vi "Upload_Balance Data_to_Server.vi"() -> ()   [LabVIEW 2015]
uses:
  Controls/Post_Process.ctl
  Globals/Meas_global.vi
panel:
  in  "millisecond multiple":dbl=100.0
  out "roll":dbl(graph)
  out "yaw":dbl(graph)
  out "side":dbl(graph)
  out "drag":dbl(graph)
  out "pitch":dbl(graph)
  out "lift":dbl(graph)
  out "appended array":dbl[](array[numeric])
  out "Monitor Speed (Hz)":dbl
  in  "stop":bool
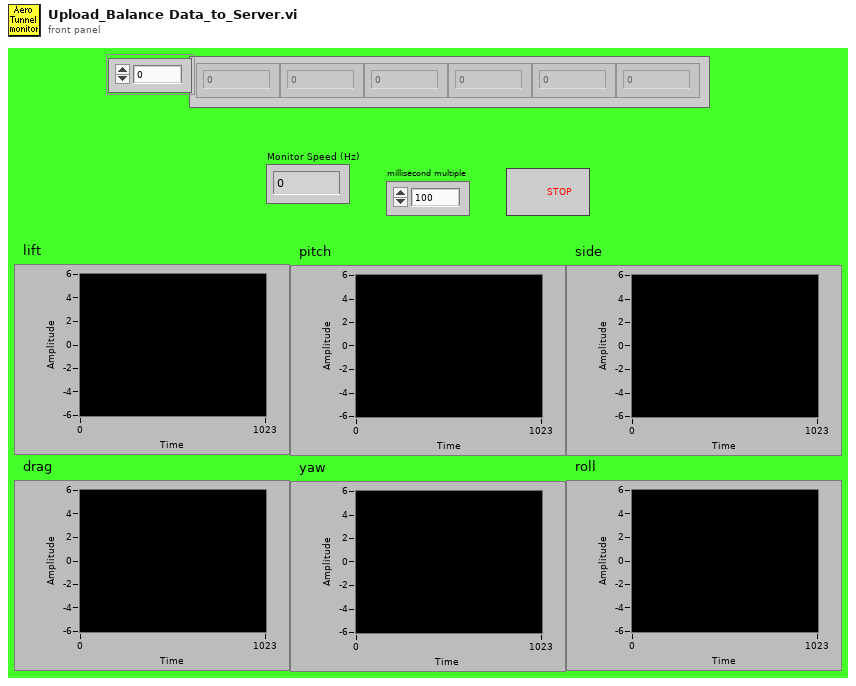
[diagram p1: front panel]
types:
  T1 = typedef "Post_Process.ctl" = enum16{"Take New Data", "Post Process Raw Data File"}
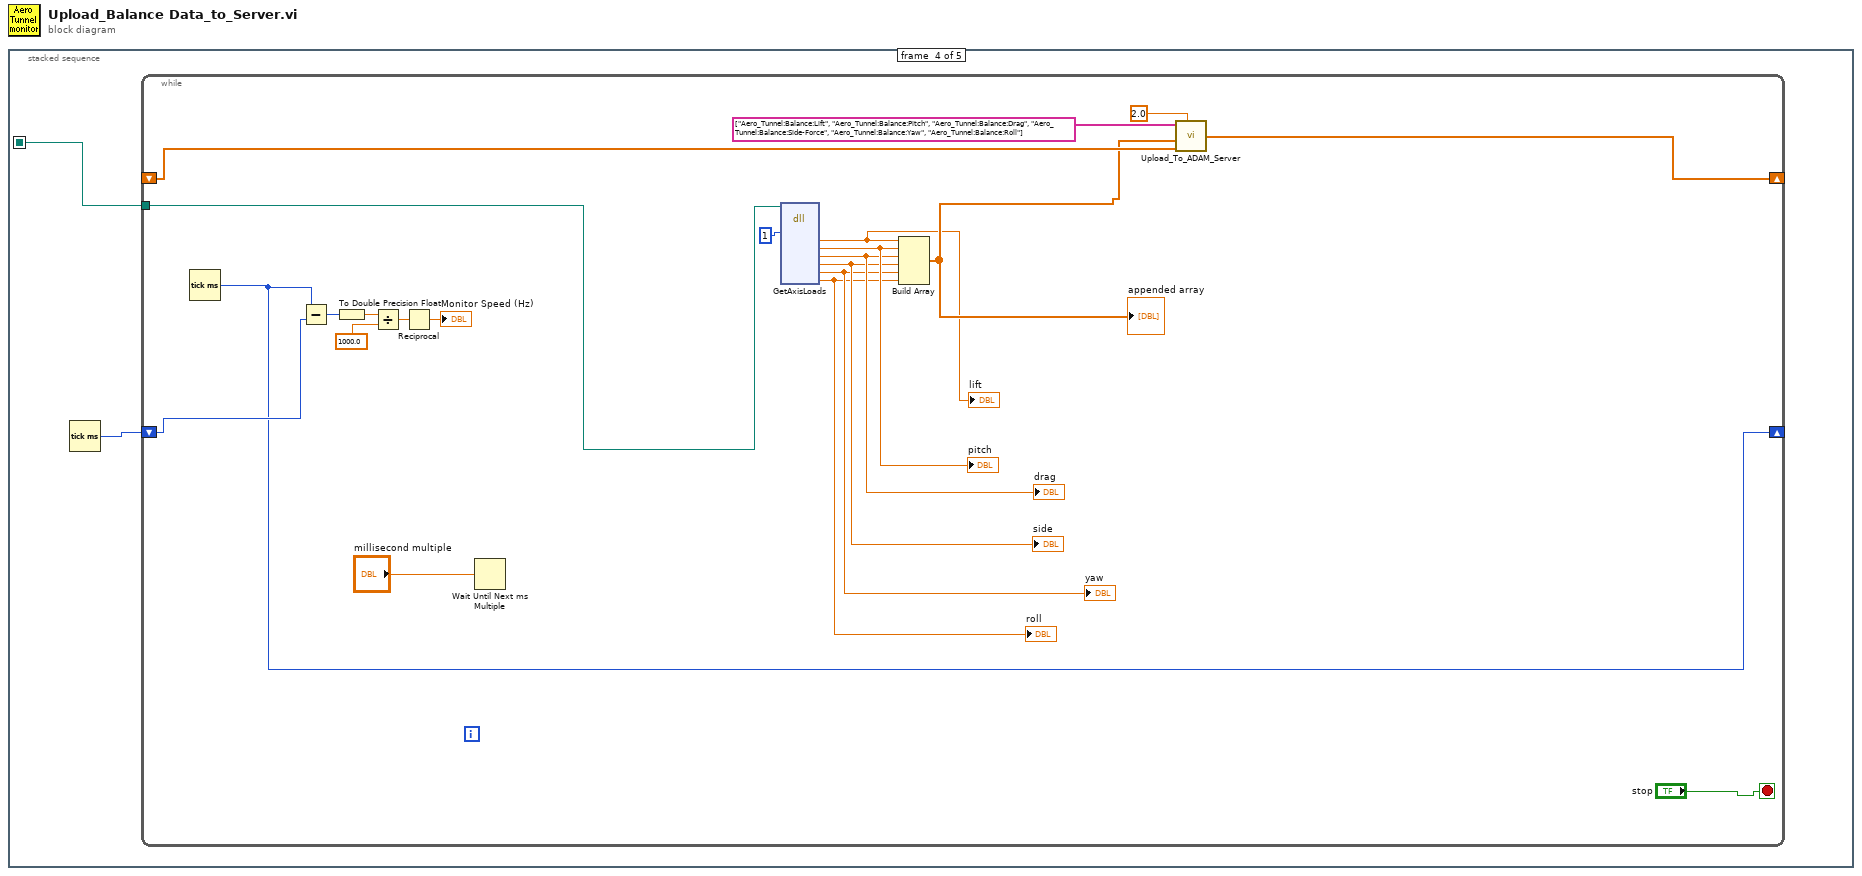
[diagram p0: block diagram]
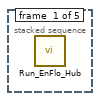
[diagram p2: hidden frame]
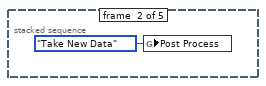
[diagram p3: hidden frame]
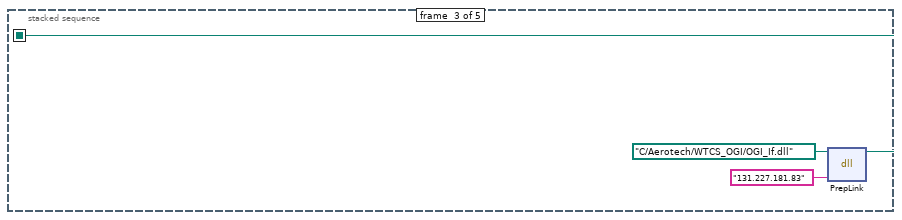
[diagram p4: hidden frame]
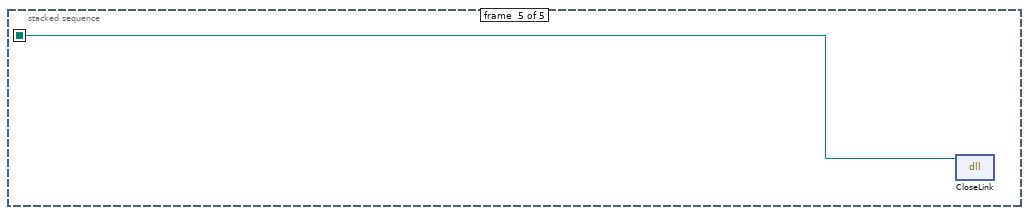
[diagram p5: hidden frame]
diagram:
  n1 = stacked-sequence {
    seq-local: [_ _ w2 _ _] -> [_ _ _ w6 w29]
    frame #0 {
      n2 = call "Run_EnFlo_Hub.vi"() -> ()  [unwired: 7 in, 1 out]
    }
    frame #1 {
      n3 = global write "Meas_global.vi" "Post Process"(Post_Process."Take New Data" ("Post Process")) -> ()
    }
    frame #2 {
      n4 = dll-call lib="C:/Aerotech/Drivers/OGI_IF.dll" fn="PrepLink"(path in=path "C:/Aerotech/WTCS_OGI/OGI_If.dll", "IPAddress"="131.227.181.83") -> (path out=w2:path)  [unwired: 2 in, 3 out]
    }
    frame #3 {
      n5 = Tick Count (ms)() -> (millisecond timer value=w5:u32)
      n6 = while {
        tunnel: w6 -> [w28]
        shift-right: [w26] -> _
        shift-left: _ -> [w27]
        shift-right: [w23] -> _
        shift-left: w5 -> [w25]
        stop <- "stop" stop-if-true
        n7 = Tick Count (ms)() -> (millisecond timer value=w23:u32)
        n8 = Subtract(x=w23, y=w25) -> (x-y=w18:u32)
        n9 = To Double Precision Float(number=w18) -> (double precision float=w14:dbl)
        n10 = Divide(x=w14, y=1000.0) -> (x/y=w16:dbl)
        n11 = Reciprocal(x=w16) -> (1/x=→"Monitor Speed (Hz)":dbl)
        n12 = Wait Until Next ms Multiple(millisecond multiple="millisecond multiple") -> ()  [unwired: 1 out]
        n13 = dll-call lib="C:/Aerotech/Drivers/OGI_IF.dll" fn="GetAxisLoads"(path in=w28, "Enable"=1) -> ("Lift"=w7:dbl, "Pitch"=w13:dbl, "Drag"=w12:dbl, "side"=w11:dbl, "Yaw"=w10:dbl, "Roll"=w9:dbl)  [unwired: 3 in, 9 out]
        "lift" <- w7
        "pitch" <- w13
        "drag" <- w12
        "side" <- w11
        "yaw" <- w10
        "roll" <- w9
        n14 = Build Array(w7, w13, w12, w11, w10, w9) -> (w19:dbl[])
        "appended array" <- w19
        n15 = call "Upload_To_ADAM_Server.vi"("Averaging Period (s)"=2.0, "Shift In"=w27, "Channel Values"=w19, "Channel Names"=string[] ["Aero_Tunnel:Balance:Lift", "Aero_Tunnel:Balance:Pitch", "Aero_Tunnel:Balance:Drag", "Aero_Tunnel:Balance:Side-Force", "Aero_Tunnel:Balance:Yaw", "Aero_Tunnel:Balance:Roll"]) -> ("Shift Out"=w26:dbl[])  [unwired: 2 in]
      }
    }
    frame #4 {
      n16 = dll-call lib="C:/Aerotech/Drivers/OGI_IF.dll" fn="CloseLink"(path in=w29) -> ()  [unwired: 2 in, 3 out]
    }
  }
